vi "ClearFaults.vi"(8 "error in (no error)":errorcluster, 11 "SoftmotionAxis in":refnum<class "SoftmotionAxis.lvclass">) -> (0 "error out":errorcluster, 3 "SoftmotionAxis out":refnum<class "SoftmotionAxis.lvclass">)   [LabVIEW 2017, in "SoftmotionAxis.lvclass"]
uses:
  SoftmotionAxis.lvclass
  <resource>/objmgr/nimcai.rc
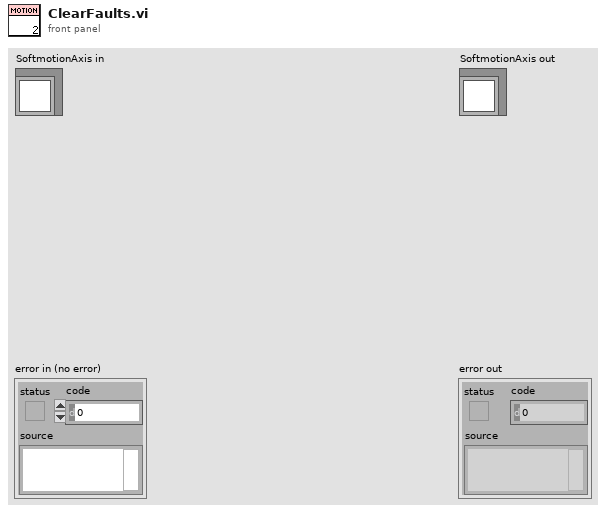
[diagram p1: front panel]
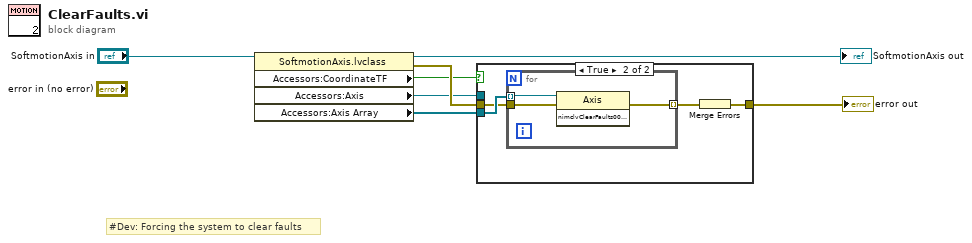
[diagram p0: block diagram]
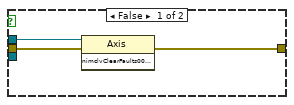
[diagram p2: hidden frame]
diagram:
  # "#Dev: Forcing the system to clear faults"
  n1 = property class="SoftmotionAxis.lvclass"(reference="SoftmotionAxis in") -> (reference out=→"SoftmotionAxis out":refnum<class "SoftmotionAxis.lvclass">, error out=w3:errorcluster, "Accessors:CoordinateTF"=w2:bool, "Accessors:Axis"=w1:refnum<k21>, "Accessors:Axis Array"=w4:refnum<k21>[])  [unwired: 1 in]
  n2 = case shown="True" w2 {
    tunnel: [w8 w14] -> w7
    tunnel: w4 -> [_ w13]
    tunnel: w3 -> [w9 w12]
    tunnel: w1 -> [w10 _]
    frame False {
      n3 = invoke class="Axis" method="nimclvClearFaults00A10001"(reference=w10, error in=w9) -> (error out=w8:errorcluster)  [unwired: 1 in, 2 out]
    }
    frame True {
      n4 = for {
        tunnel: w13 -> [w17] mode=indexing
        tunnel: w12 -> [w16]
        tunnel: [w15] -> w11 mode=indexing
        n5 = invoke class="Axis" method="nimclvClearFaults00A10001"(reference=w17, error in=w16) -> (error out=w15:errorcluster)  [unwired: 1 in, 2 out]
      }
      n6 = Merge Errors(w11) -> (w14:errorcluster)
    }
  }
  "error out" <- w7
